vi "save protocol notes.vi"   [LabVIEW 2012]
doc: "SciScan 1.0 151216"
uses:
  GFG/GFGpathGet.vi
  GFG/GFG library.lvlib
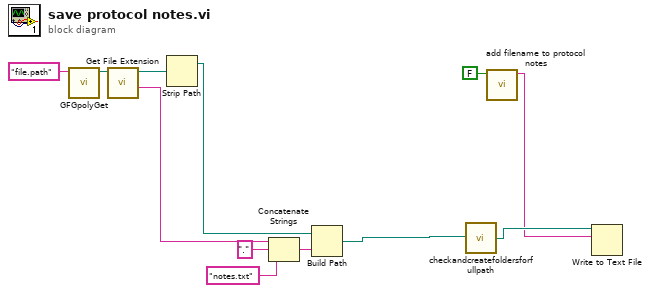
[diagram p0: block diagram]
diagram:
  n1 = call-poly "GFGpolyGet.vi"("Variable Name in"="file.path") -> ("Path"=w7:path)  [unwired: 8 in, 2 out]
  n2 = call <vilib>:"Get File Extension.vi"("file"=w7) -> ("filename without extension"=w6:string)  [unwired: 7 in, 3 out]
  n3 = Strip Path(path=w7) -> (stripped path=w5:path)  [unwired: 1 out]
  n4 = Concatenate Strings(w6, "." ("string"), "notes.txt" ("string")) -> (w4:string)
  n5 = Build Path(base path=w5, name or relative path=w4) -> (appended path=w11:path)
  n6 = call "checkandcreatefoldersforfullpath.vi"("Path IN"=w11) -> ("Path OUT"=w3:path)  [unwired: 4 in]
  n7 = call "add filename to protocol notes.vi"("rec start/end (T is start)"=FALSE) -> ("protocol.notes out"=w1:string)  [unwired: 10 in]
  n8 = Write to Text File(file (use dialog)=w3, text=w1) -> ()  [unwired: 2 in, 3 out]
